vi "FetchScans.vi"(8 "error in (no error)":errorcluster, 11 "Experiment in":refnum<class "Experiment.lvclass">) -> (0 "error out":errorcluster, 2 "data":string[][](array[string]), 3 "Experiment out":refnum<class "Experiment.lvclass">)   [LabVIEW 2016, in "Experiment.lvclass"]
uses:
  Experiment.lvclass
  Experiment.lvclass/Experiment.ctl
  Database/Database.lvclass
panel:
  out "columns":string[](array[string])
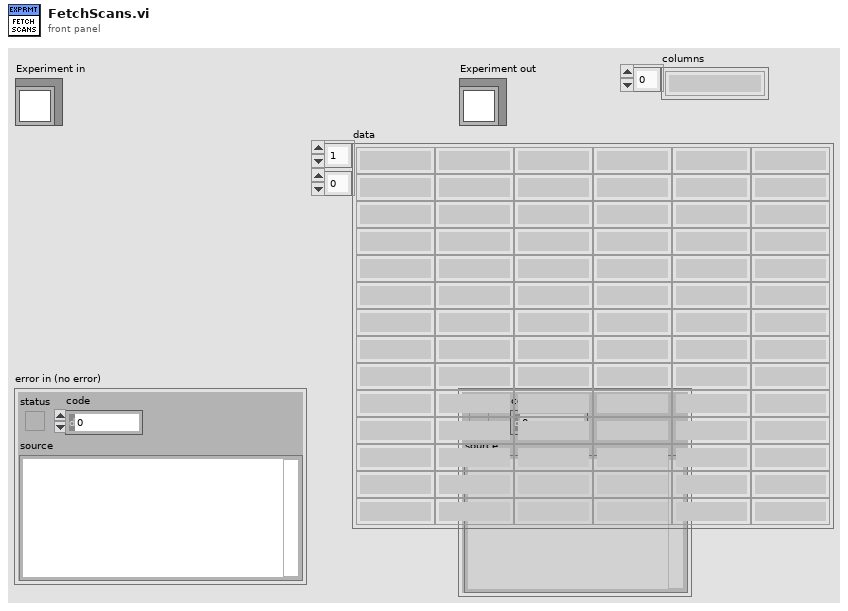
[diagram p1: front panel]
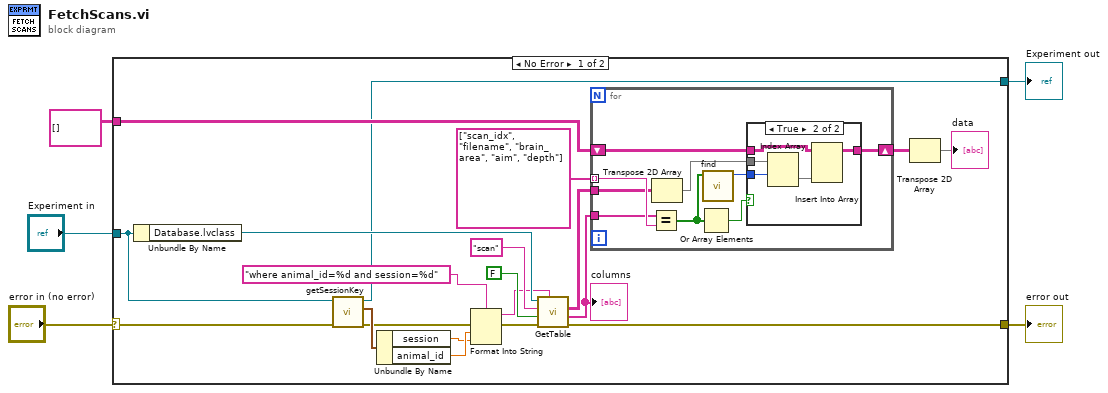
[diagram p0: block diagram]
diagram:
  n1 = case shown="No Error" "error in (no error)" {
    selector: "error in (no error)" -> [w13 w42]
    tunnel: [w24 w42] -> w4
    tunnel: [w14 w41] -> w2
    tunnel: "Experiment in" -> [w15 w41]
    tunnel: string[][] [] ("data") -> [w19 _]
    frame No Error {
      n2 = Unbundle By Name(w15) -> ("Database.lvclass"=w25:refnum<class "Database.lvclass">)
      n3 = call-dynamic "getSessionKey.vi"("error in (no error)"=w13, "Experiment in"=w15) -> ("error out"=w7:errorcluster, "Session Key"=w11:cluster{"session":dbl, "animal_id":dbl}, "Experiment out"=w14:refnum<class "Experiment.lvclass">)  [unwired: 7 in]
      n4 = Unbundle By Name(w11) -> ("session"=w9:dbl, "animal_id"=w10:dbl)
      n5 = Format Into String(format string="where animal_id=%d and session=%d", error in=w7, w10, w9) -> (resulting string=w8:string, error out=w6:errorcluster)  [unwired: 1 in]
      n6 = call-dynamic "GetTable.vi"("condition"=w8, "error in (no error)"=w6, "Primary"=FALSE, "table"="scan", "Database in"=w25) -> ("error out"=w24:errorcluster, "columns"=w20:string[], "data"=w18:string[][])  [unwired: 3 in, 1 out]
      "columns" <- w20
      n7 = for {
        tunnel: string[] ["scan_idx", "filename", "brain_area", "aim", "depth"] -> [w34] mode=indexing
        tunnel: w20 -> [w33]
        tunnel: w18 -> [w29]
        shift-right: [w31] -> w17
        shift-left: w19 -> [w32]
        n8 = Equal?(x=w33, y=w34) -> (x = y?=w27:bool[])
        n9 = Transpose 2D Array(2D array=w29) -> (transposed array=w28:string[][])
        n10 = Or Array Elements(Boolean array=w27) -> (logical OR=w30:bool)
        n11 = call "find.vi"("Array"=w27) -> ("Index"=w26:i32)  [unwired: 10 in]
        n12 = case shown="True" w30 {
          tunnel: w28 -> [_ w38]
          tunnel: w26 -> [_ w37]
          tunnel: w32 -> [w35 w40]
          tunnel: [w35 w39] -> w31
          frame False {
          }
          frame True {
            n13 = Index Array(array=w38, index (row)=w37) -> (element=w36:string[])  [unwired: 1 in]
            n14 = Insert Into Array(array=w40, new element=w36) -> (w39:string[][])  [unwired: 2 in]
          }
        }
      }
      n15 = Transpose 2D Array(2D array=w17) -> (transposed array=→"data":string[][])
    }
    frame Error {
    }
  }
  "error out" <- w4
  "Experiment out" <- w2
